vi "Get Name.vi"(10 "Include Extra Info":bool, 11 "CIFPluginManager in":refnum<class "CIFPluginManager.lvclass">) -> (3 "Name":string)   [LabVIEW 2021, in "CIFPluginManager.lvclass"]
uses:
  CIFPluginManager.lvclass
  CIFPluginManager.lvclass/CIFPluginManager.ctl
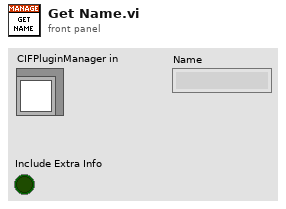
[diagram p1: front panel]
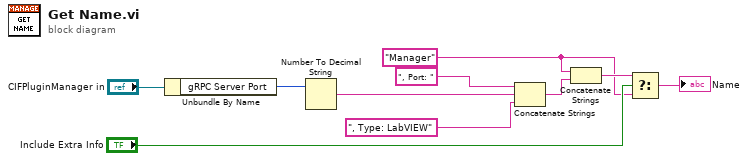
[diagram p0: block diagram]
diagram:
  w1 = "Manager" ("message")
  n1 = Unbundle By Name("CIFPluginManager in") -> ("gRPC Server Port"=w10:i32)
  n2 = Number To Decimal String(number=w10) -> (decimal integer string=w9:string)  [unwired: 1 in]
  n3 = Concatenate Strings(", Port: " ("message"), w9, ", Type: LabVIEW" ("message")) -> (w6:string)
  n4 = Concatenate Strings(w1, w6) -> (w5:string)
  n5 = Select(t=w5, s="Include Extra Info", f=w1) -> (s? t:f=→"Name":string)
